vi "Calibration Calibrate (Set).vi"(6 "ISOBUS address":T3=-1 caption="ISOBUS address (-1)", 8 "error in":errorcluster, 11 "Mercury Reference In":T4) -> (0 "error out":errorcluster, 2 "Response":T1, 3 "Mercury Reference Out":T4, 4 "Valid?":T2)   [LabVIEW 2013, in "Mercury iXX.lvlib" / "Pressure.lvlib"]
doc: "Set the current calibration offset for the selected pressure device."
uses:
  Pressure.lvlib
  Mercury iXX.lvlib
  Private/Controls/Command Verbs.ctl
  Controls/Response String.ctl
  Controls/Is Valid LED.ctl
  Controls/Comms Transport Layer.ctl
  Controls/Mercury Reference.ctl
  Controls/ISOBus Address.ctl
  Private/Controls/Query Dynamic Reference.ctl
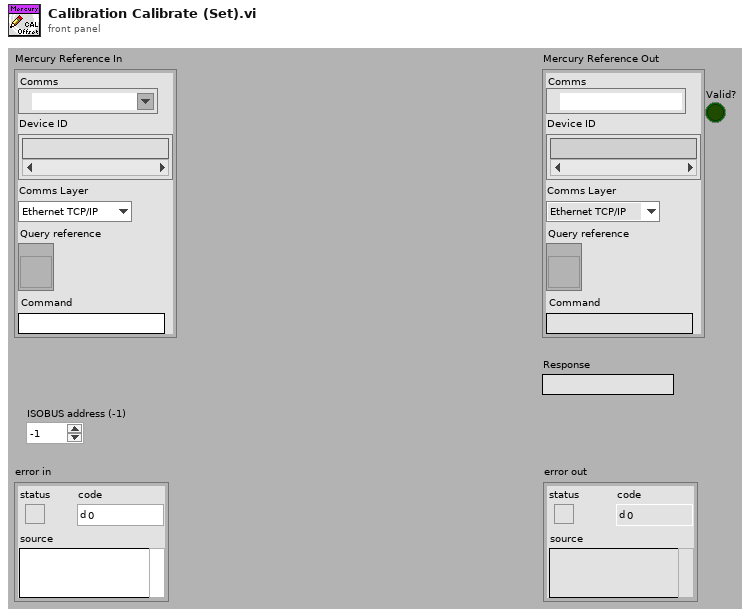
[diagram p1: front panel]
types:
  T1 = typedef "Mercury iXX.lvlib/Response String.ctl" = string
  T2 = typedef "Mercury iXX.lvlib/Is Valid LED.ctl" = bool
  T3 = typedef "Mercury iXX.lvlib/ISOBus Address.ctl" = i32
  T4 = typedef "Mercury iXX.lvlib/Mercury Reference.ctl" = cluster{"Comms":refnum<visa-resource-name>, "Device ID":string[], "Comms Layer":T5, "Command":string, "Query reference":T6}
  T5 = typedef "Mercury iXX.lvlib/Comms Transport Layer.ctl" = enum16{"Ethernet TCP/IP", "USB", "ISOBus - RS-232", "GPIB"}
  T6 = typedef "Mercury iXX.lvlib/Query Dynamic Reference.ctl" = refnum<vi>
  T7 = typedef "Mercury iXX.lvlib/Command Verbs.ctl" = string
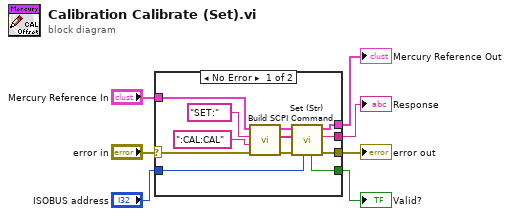
[diagram p0: block diagram]
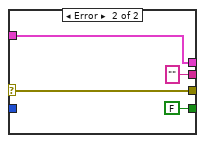
[diagram p2: hidden frame]
diagram:
  n1 = case shown="No Error" "error in" {
    selector: "error in" -> [w8 w23]
    tunnel: [w14 w23] -> w7
    tunnel: "ISOBUS address" -> [w13 _]
    tunnel: [w12 T2 FALSE ("Valid?")] -> w5
    tunnel: [w11 T1 "" ("Response")] -> w4
    tunnel: [w10 w22] -> w3
    tunnel: "Mercury Reference In" -> [w9 w22]
    frame No Error {
      n2 = call "Build SCPI Command.vi"("error in"=w8, "Noun(s)"=":CAL:CAL" ("Command"), "Verb"=T7 "SET:", "Mercury Reference In"=w9) -> ("error out"=w19:errorcluster, "SCPI Message(s)"=w18:string[], "Mercury Reference Out"=w17:T4)  [unwired: 5 out]
      n3 = call "Set (Str).vi"("ISOBUS address"=w13, "error in"=w19, "SCPI Message(s)"=w18, "Mercury Reference In"=w17) -> ("error out"=w14:errorcluster, "Response"=w11:T1, "Mercury Reference Out"=w10:T4, "Valid?"=w12:T2)  [unwired: 1 in, 3 out]
    }
    frame Error {
    }
  }
  "Mercury Reference Out" <- w3
  "error out" <- w7
  "Valid?" <- w5
  "Response" <- w4
